vi "FTW-Scripter-Core_Process.vi"(0 "FTW Actor Instance Configuration":string="{\n  \"Identity\": \"FTW Scripter\",\n  \"InboxAddress\": \"inproc://*\",\n  \"LoggerAddress\": \"\",\n  \"Connections\": {},\n  \"Publishers\": {\n    \"ScripterStatus\": \"inproc://*\"\n  },\n  \"Subscriptions\": {},\n  \"Step Name Dictionary\": {},\n  \"Refresh Period\": 0.1\n}", 11 "ErrorIn":errorcluster) -> (15 "Error":errorcluster)   [LabVIEW 2015, in "FTW-Scripter-Core.lvclass"]
uses:
  FTW-Scripter-Core.lvclass
  source/actor/Instance/FTW-ActorInstance.lvclass
  source/actor/Message/Request/FTW-Message-IncomingRequest.lvclass
  source/actor/Message/Base/FTW-Message.lvclass
  source/actor/Instance-Extended/FTW-ActorExtended.lvclass
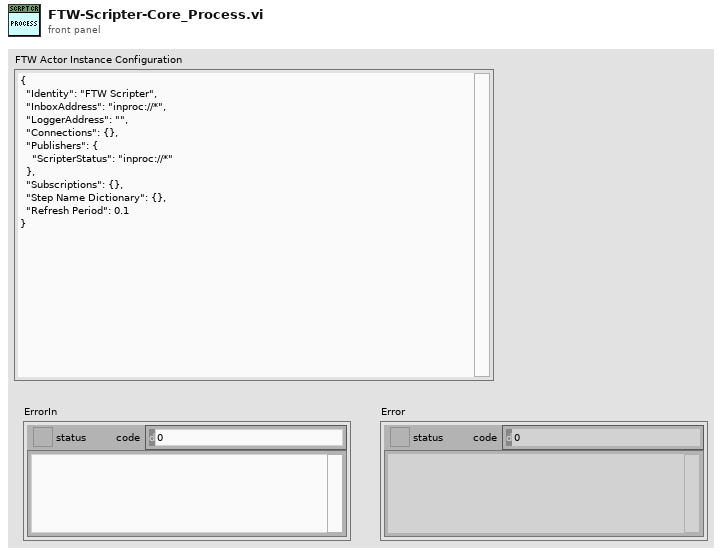
[diagram p1: front panel]
types:
  T1 = cluster{"Incoming Requests":refnum<event-registration>, "Local Messages":refnum<event-registration>, "Subscriber Registration":refnum<event-registration>}
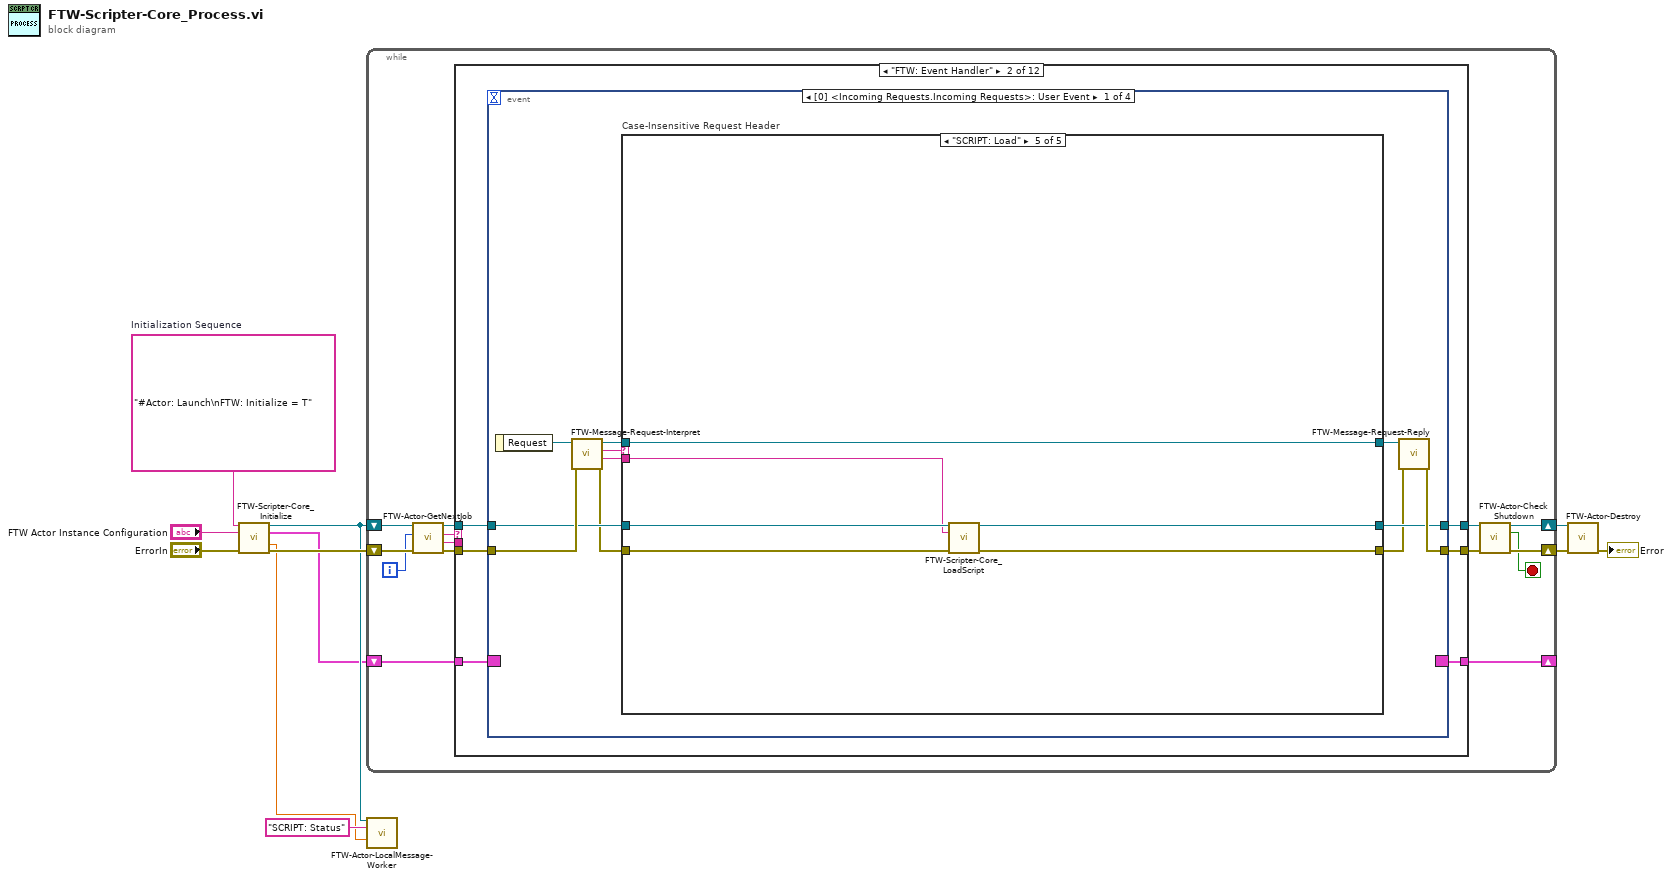
[diagram p0: block diagram]
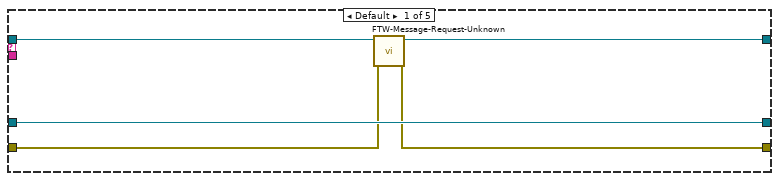
[diagram p3: hidden frame]
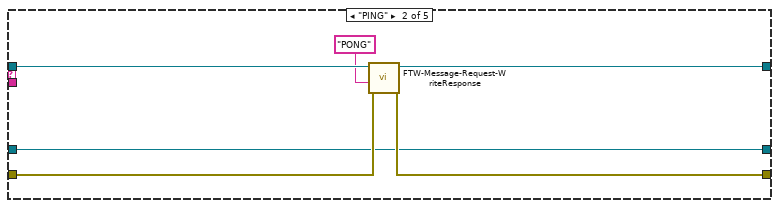
[diagram p4: hidden frame]
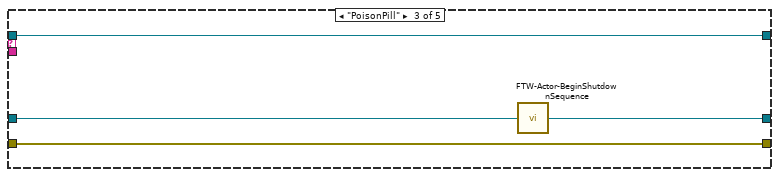
[diagram p5: hidden frame]
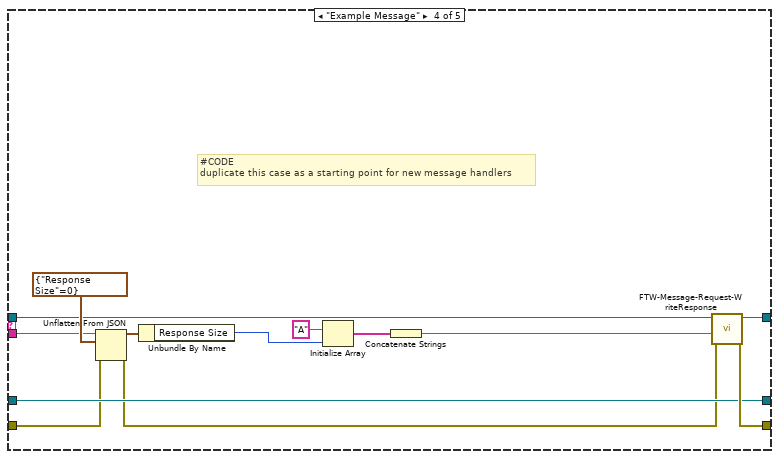
[diagram p6: hidden frame]
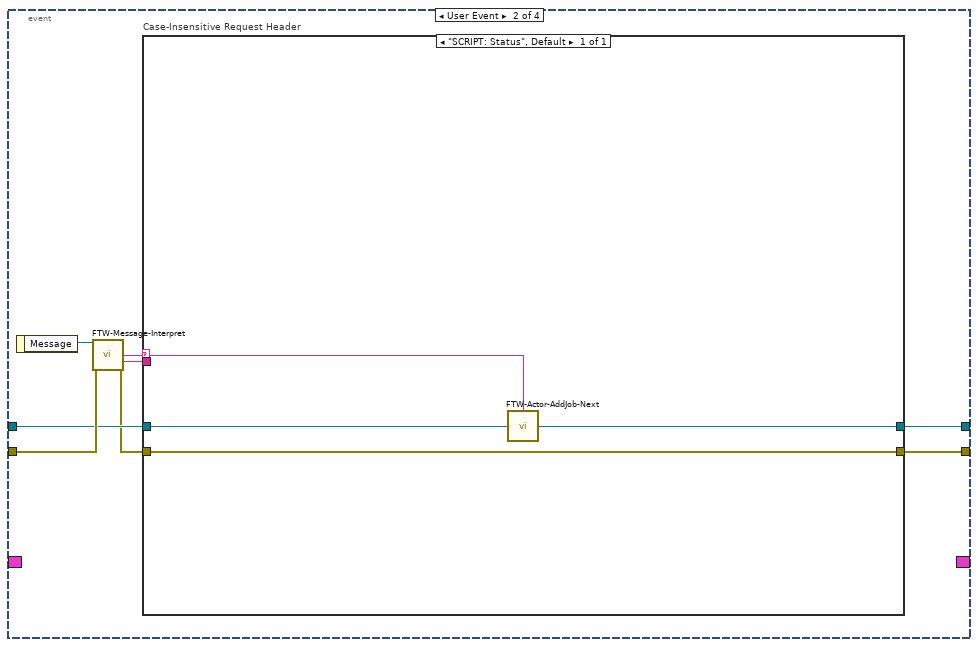
[diagram p7: hidden frame]
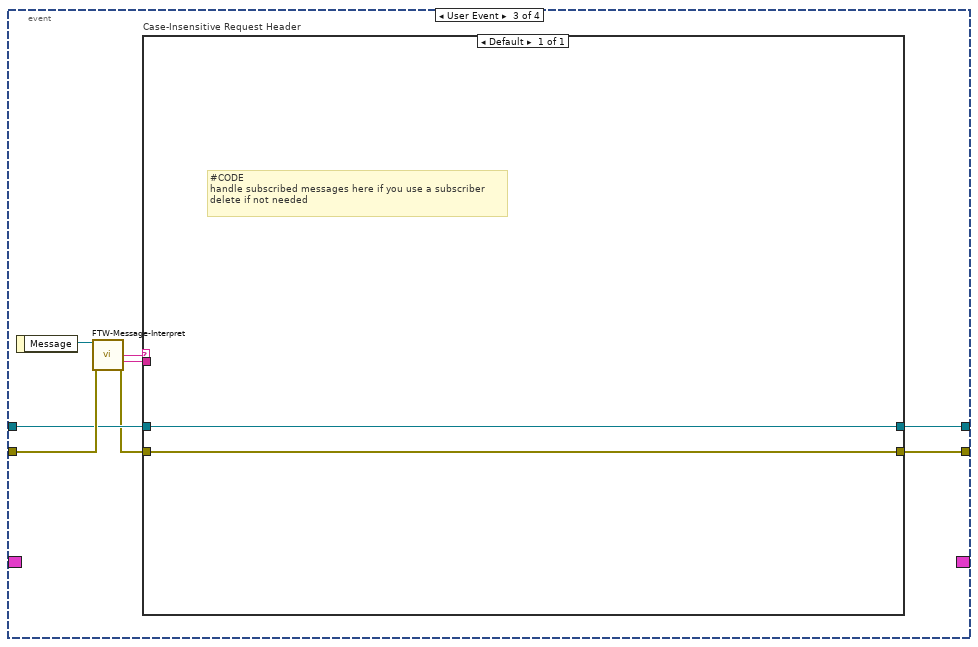
[diagram p8: hidden frame]
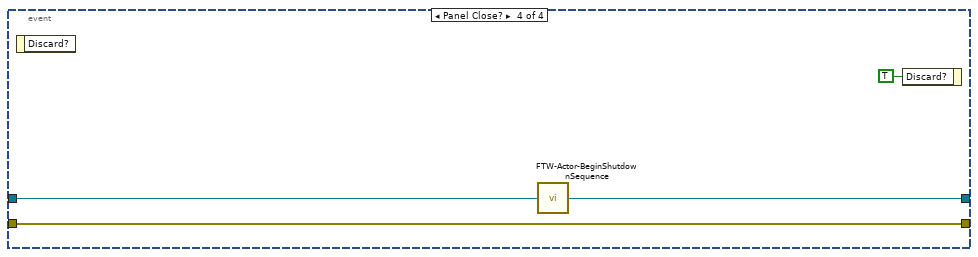
[diagram p9: hidden frame]
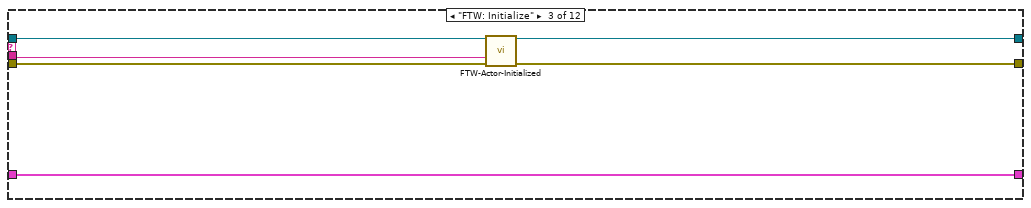
[diagram p10: hidden frame]
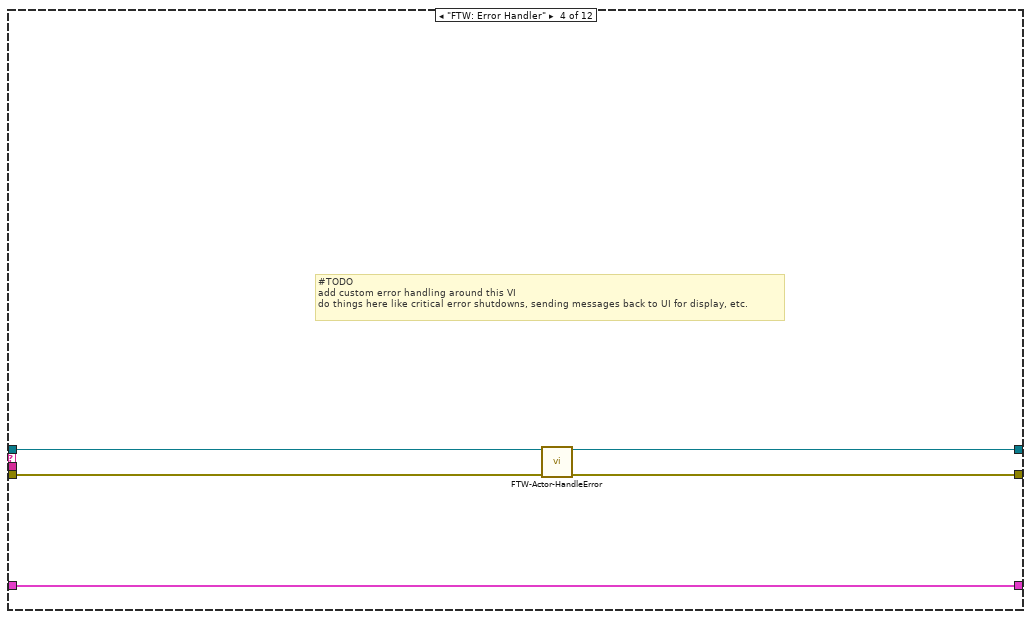
[diagram p11: hidden frame]
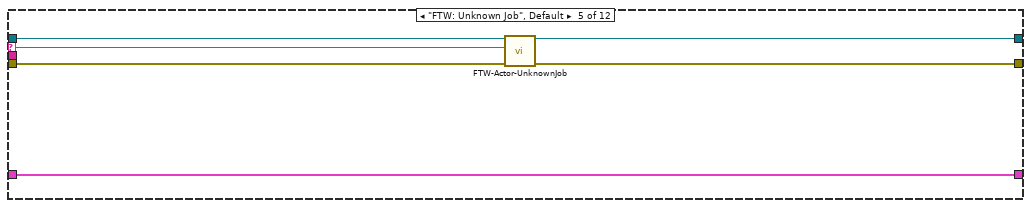
[diagram p12: hidden frame]
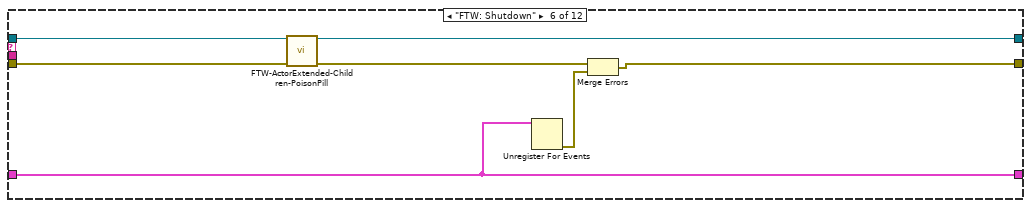
[diagram p13: hidden frame]
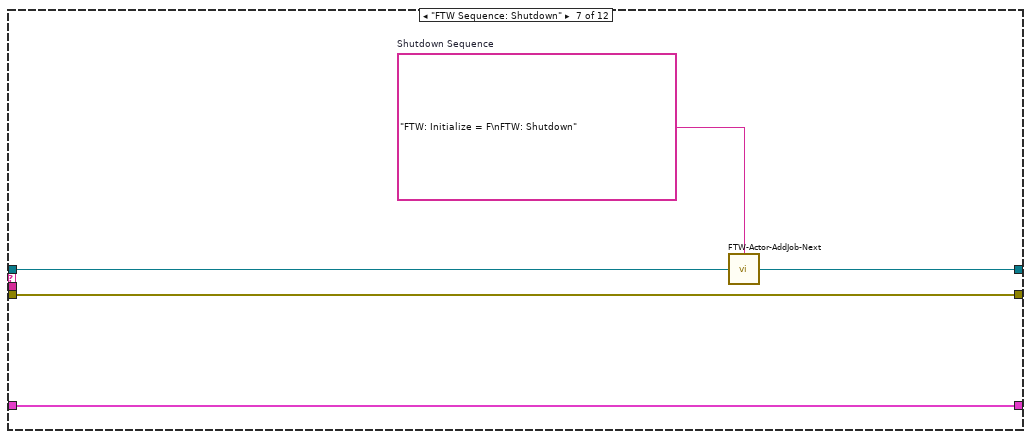
[diagram p14: hidden frame]
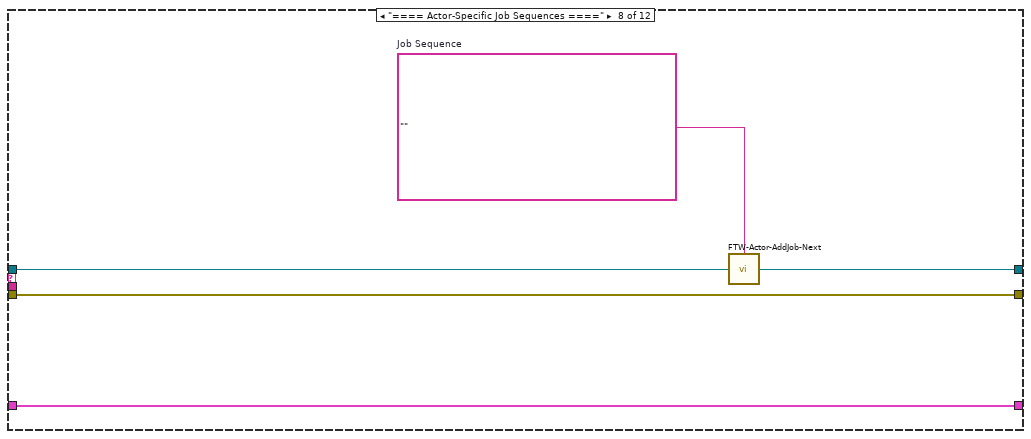
[diagram p15: hidden frame]
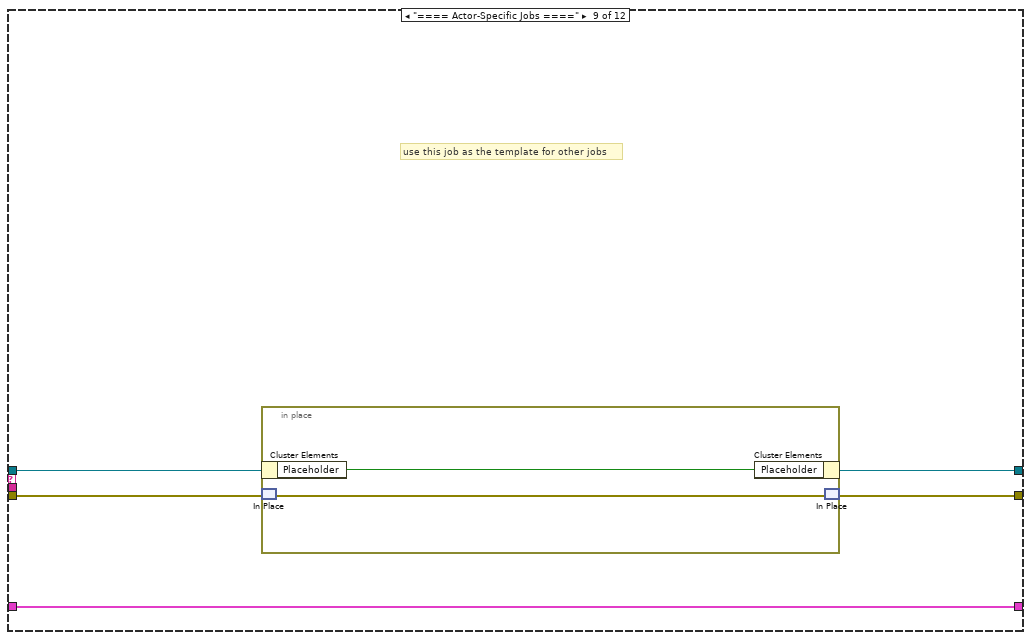
[diagram p16: hidden frame]
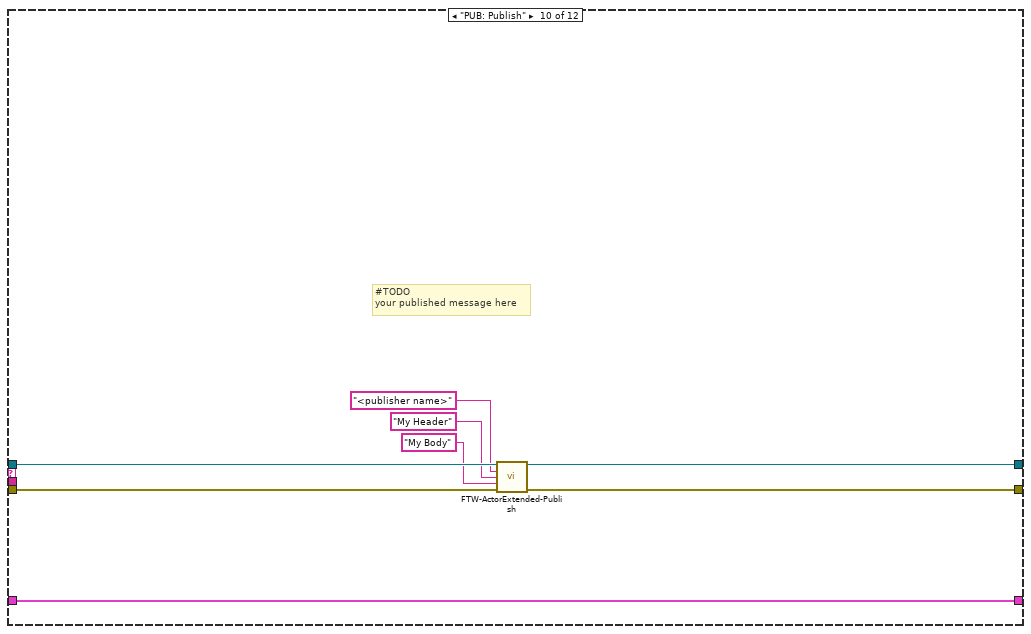
[diagram p17: hidden frame]
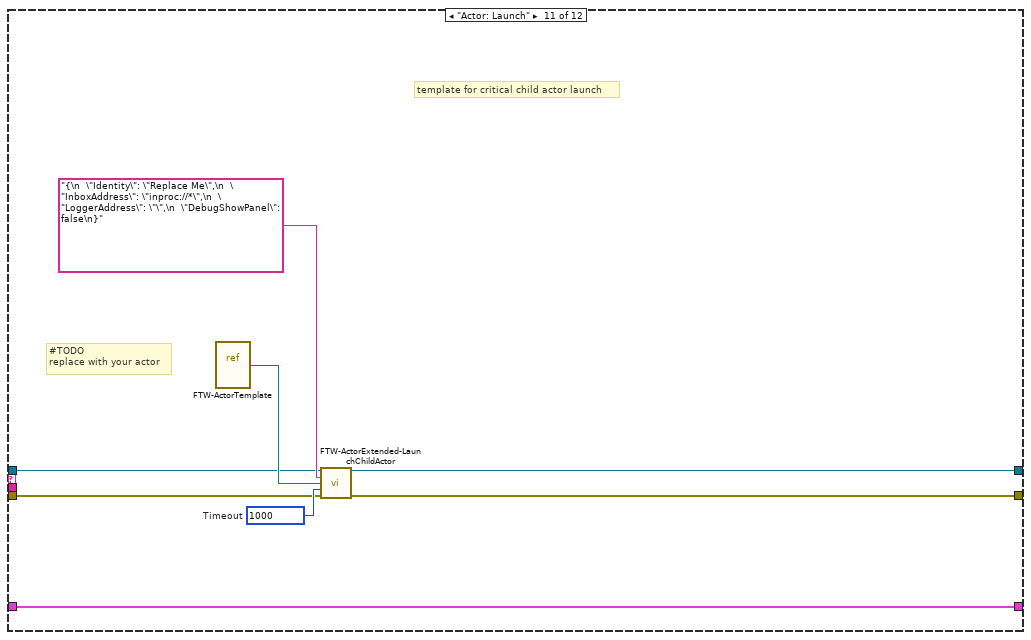
[diagram p18: hidden frame]
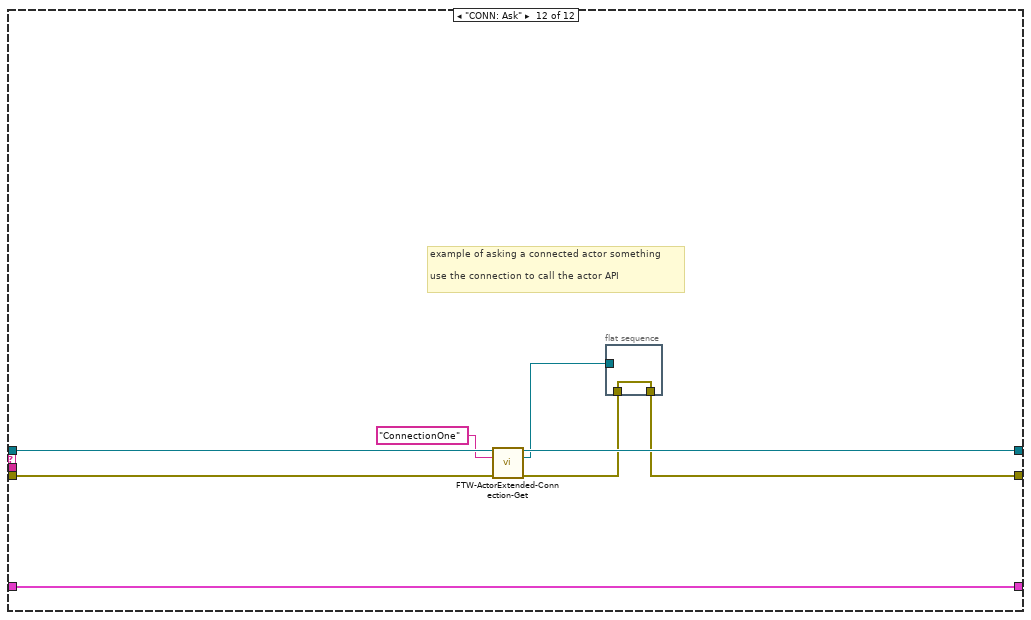
[diagram p19: hidden frame]
diagram:
  w7 = "#Actor: Launch\nFTW: Initialize = T"  # Initialization Sequence
  n1 = call "FTW-Scripter-Core_Initialize.vi"("Initialization Sequence"=w7, "FTW Actor Instance Configuration"="FTW Actor Instance Configuration", "error in (no error)"="ErrorIn") -> ("Actor Template-Core out"=w3:refnum<class "FTW-Scripter-Core.lvclass">, "Event Refnums"=w1:T1, "Refresh Period"=w2:dbl, "error out"=w8:errorcluster)  [unwired: 9 in]
  n2 = while {
    shift-right: [w15] -> w10
    shift-left: w8 -> [w22]
    shift-right: [w12] -> _
    shift-left: w1 -> [w25]
    shift-right: [w17] -> w11
    shift-left: w3 -> [w24]
    i -> [w13]
    stop <- w14 stop-if-true
    n3 = call "FTW-Actor-GetNextJob.vi"("error in"=w22, "Jobs Performed"=w13, "FTW Actor Instance"=w24) -> ("error out"=w21:errorcluster, "Job Data"=w19:string, "Job Name"=w20:string, "FTW Actor Instance out"=w23:refnum<class "FTW-Scripter-Core.lvclass">)  [unwired: 5 in]
    n4 = case shown="\"FTW: Event Handler\"" w20 {
      selector: w20 -> [_ _ _ _ w117 _ _ _ _ _ _ _]
      tunnel: [w27 w34 w108 w112 w120 w128 w133 w138 w142 w152 w157 w163] -> w16
      tunnel: w21 -> [w27 w33 w110 w114 w121 w129 w133 w138 w143 w153 w158 w169]
      tunnel: w25 -> [w28 w29 w111 w116 w122 w126 w134 w139 w144 w154 w162 w170]
      tunnel: [w28 w32 w111 w116 w122 w126 w134 w139 w144 w154 w162 w170] -> w12
      tunnel: w19 -> [_ _ w106 _ _ _ _ _ _ _ _ _]
      tunnel: [w26 w31 w109 w113 w118 w123 w131 w136 w140 w150 w155 w167] -> w18
      tunnel: w23 -> [w26 w30 w107 w115 w119 w124 w132 w137 w141 w151 w156 w168]
      frame "==== Featherweight Framework Jobs ====" {
      }
      frame "FTW: Event Handler" {
        n5 = event shown="[0] <Incoming Requests.Incoming Requests>: User Event" {
          selector: w29 -> [_ _ _ _]
          dyn-events: [_ _ _ _] -> w32
          timeout: _ -> [_ _ _ _]
          tunnel: [w44 w82 w94 w104] -> w34
          tunnel: w33 -> [w43 w86 w98 w104]
          tunnel: [w38 w83 w95 w102] -> w31
          tunnel: w30 -> [w42 w85 w97 w103]
          event User Event {
            n6 = event-data() -> ("Request"=w45:refnum<class "FTW-Message-IncomingRequest.lvclass">)  [unwired: 1 in]
            n7 = call "FTW-Message-Request-Interpret.vi"("error in"=w43, "FTW Incoming Request"=w45) -> ("error out"=w41:errorcluster, "Request Body"=w35:string, "Request Header"=w39:string, "FTW Incoming Request out"=w40:refnum<class "FTW-Message-IncomingRequest.lvclass">)  [unwired: 6 in]
            n8 = case "Case-Insensitive Request Header" shown="\"SCRIPT: Load\"" w39 {
              tunnel: [w48 w54 w59 w73 w75] -> w37
              tunnel: w41 -> [w49 w55 w59 w62 w76]
              tunnel: [w50 w53 w60 w71 w77] -> w38
              tunnel: w42 -> [w50 w53 w58 w71 w78]
              tunnel: w40 -> [w47 w56 w57 w63 w79]
              tunnel: [w46 w52 w57 w72 w79] -> w36
              tunnel: w35 -> [_ _ _ w61 w74]
              frame Default {
                n9 = call "FTW-Message-Request-Unknown.vi"("error in"=w49, "FTW Incoming Request"=w47) -> ("error out"=w48:errorcluster, "FTW Incoming Request Out"=w46:refnum<class "FTW-Message-IncomingRequest.lvclass">)  [unwired: 8 in]
              }
              frame "PING" {
                n10 = call "FTW-Message-Request-WriteResponse.vi"("error in"=w55, "Response Body"="PONG" ("Response Header"), "FTW Incoming Request"=w56) -> ("error out"=w54:errorcluster, "FTW Incoming Request out"=w52:refnum<class "FTW-Message-IncomingRequest.lvclass">)  [unwired: 7 in]
              }
              frame "PoisonPill" {
                n11 = call "FTW-Actor-BeginShutdownSequence.vi"("FTW Actor Instance"=w58) -> ("FTW Actor Instance out"=w60:refnum<class "FTW-Scripter-Core.lvclass">)  [unwired: 3 in]
              }
              frame "Example Message" {
                # "#CODE\nduplicate this case as a starting point for new message handlers"
                n12 = Unflatten From JSON(JSON string=w61, type and defaults=cluster{"Response Size":i32} {"Response Size"=0}, error in (no error)=w62) -> (value=w68:cluster{"Response Size":i32}, error out=w70:errorcluster)  [unwired: 4 in]
                n13 = Unbundle By Name(w68) -> ("Response Size"=w67:i32)
                n14 = Initialize Array("A", w67) -> (w65:string[])
                n15 = Concatenate Strings(w65) -> (w64:string)
                n16 = call "FTW-Message-Request-WriteResponse.vi"("error in"=w70, "Response Body"=w64, "FTW Incoming Request"=w63) -> ("error out"=w73:errorcluster, "FTW Incoming Request out"=w72:refnum<class "FTW-Message-IncomingRequest.lvclass">)  [unwired: 7 in]
              }
              frame "SCRIPT: Load" {
                n17 = call "FTW-Scripter-Core_LoadScript.vi"("FTW-Scripter-Core In"=w78, "Script"=w74, "error in"=w76) -> ("FTW-Scripter-Core Out"=w77:refnum<class "FTW-Scripter-Core.lvclass">, "error out"=w75:errorcluster)  [unwired: 11 in]
              }
            }
            n18 = call "FTW-Message-Request-Reply.vi"("FTW: Reply Error"=w37, "FTW Incoming Request"=w36) -> ("error out"=w44:errorcluster)  [unwired: 8 in, 1 out]
          }
          event User Event {
            n19 = event-data() -> ("Message"=w87:refnum<class "FTW-Message.lvclass">)  [unwired: 1 in]
            n20 = call-dynamic "FTW-Message-Interpret.vi"("FTW Message"=w87, "error in"=w86) -> ("Message Header"=w81:string, "Message Body"=w80:string, "error out"=w84:errorcluster)  [unwired: 9 in, 2 out]
            n21 = case "Case-Insensitive Request Header" shown="\"SCRIPT: Status\", Default" w81 {
              selector: w81 -> [w88]
              tunnel: [w90] -> w82
              tunnel: w84 -> [w90]
              tunnel: [w89] -> w83
              tunnel: w85 -> [w91]
              tunnel: w80 -> [_]
              frame "SCRIPT: Status", Default {
                n22 = call "FTW-Actor-AddJob-Next.vi"("Add Next in Job Queue"=w88, "FTW Actor Instance"=w91) -> ("FTW Actor Instance out"=w89:refnum<class "FTW-Scripter-Core.lvclass">)  [unwired: 2 in]
              }
            }
          }
          event User Event {
            n23 = event-data() -> ("Message"=w99:refnum<class "FTW-Message.lvclass">)  [unwired: 1 in]
            n24 = call-dynamic "FTW-Message-Interpret.vi"("FTW Message"=w99, "error in"=w98) -> ("Message Header"=w93:string, "Message Body"=w92:string, "error out"=w96:errorcluster)  [unwired: 9 in, 2 out]
            n25 = case "Case-Insensitive Request Header" shown="Default" w93 {
              tunnel: [w100] -> w94
              tunnel: w96 -> [w100]
              tunnel: [w101] -> w95
              tunnel: w97 -> [w101]
              tunnel: w92 -> [_]
              frame Default {
                # "#CODE\nhandle subscribed messages here if you use a subscriber\ndelete if not needed"
              }
            }
          }
          event Panel Close? {
            n26 = event-data() -> ()  [unwired: 1 in, 1 out]
            n27 = call "FTW-Actor-BeginShutdownSequence.vi"("FTW Actor Instance"=w103) -> ("FTW Actor Instance out"=w102:refnum<class "FTW-Scripter-Core.lvclass">)  [unwired: 3 in]
            n28 = event-data("Discard?"=TRUE) -> ()  [unwired: 1 in, 1 out]
          }
        }
      }
      frame "FTW: Initialize" {
        n29 = call-dynamic "FTW-Actor-Initialized.vi"("FTW Actor Instance"=w107, "Positive Init?"=w106, "error in"=w110) -> ("FTW Actor Instance out"=w109:refnum<class "FTW-Scripter-Core.lvclass">, "error out"=w108:errorcluster)  [unwired: 11 in]
      }
      frame "FTW: Error Handler" {
        # "#TODO\nadd custom error handling around this VI\ndo things here like critical error shutdowns, sending messages back to UI for display, etc."
        n30 = call-dynamic "FTW-Actor-HandleError.vi"("FTW Actor Instance"=w115, "error in"=w114) -> ("FTW Actor Instance out"=w113:refnum<class "FTW-Scripter-Core.lvclass">, "error out"=w112:errorcluster)  [unwired: 10 in, 2 out]
      }
      frame "FTW: Unknown Job", Default {
        n31 = call-dynamic "FTW-Actor-UnknownJob.vi"("FTW Actor Instance"=w119, "Unknown Job"=w117, "error in"=w121) -> ("FTW Actor Instance out"=w118:refnum<class "FTW-Scripter-Core.lvclass">, "error out"=w120:errorcluster)  [unwired: 11 in]
      }
      frame "FTW: Shutdown" {
        n32 = call "FTW-ActorExtended-Children-PoisonPill.vi"("FTW-ActorExtended In"=w124, "error in"=w129) -> ("FTW-ActorExtended Out"=w123:refnum<class "FTW-Scripter-Core.lvclass">, "error out"=w125:errorcluster)  [unwired: 12 in]
        n33 = Unregister For Events(event registration refnum=w126) -> (error out=w127:errorcluster)  [unwired: 1 in]
        n34 = Merge Errors(w125, w127) -> (w128:errorcluster)
      }
      frame "FTW Sequence: Shutdown" {
        w130 = "FTW: Initialize = F\nFTW: Shutdown"  # Shutdown Sequence
        n35 = call "FTW-Actor-AddJob-Next.vi"("Add Next in Job Queue"=w130, "FTW Actor Instance"=w132) -> ("FTW Actor Instance out"=w131:refnum<class "FTW-Scripter-Core.lvclass">)  [unwired: 2 in]
      }
      frame "==== Actor-Specific Job Sequences ====" {
        w135 = ""  # Job Sequence
        n36 = call "FTW-Actor-AddJob-Next.vi"("Add Next in Job Queue"=w135, "FTW Actor Instance"=w137) -> ("FTW Actor Instance out"=w136:refnum<class "FTW-Scripter-Core.lvclass">)  [unwired: 2 in]
      }
      frame "==== Actor-Specific Jobs ====" {
        # "use this job as the template for other jobs"
        n37 = in-place {
          n38 = in-place-cluster #1(w141) -> ("Placeholder"=w145:bool)
          n39 = in-place-match #2(w143) -> (w146:errorcluster)
          n40 = in-place-cluster #1("Placeholder"=w145) -> (w140:refnum<class "FTW-Scripter-Core.lvclass">)
          n41 = in-place-match #2(w146) -> (w142:errorcluster)
        }
      }
      frame "PUB: Publish" {
        # "#TODO\nyour published message here"
        n42 = call "FTW-ActorExtended-Publish.vi"("FTW-ActorExtended In"=w151, "Publisher Name"="<publisher name>", "Message Header"="My Header" ("Header"), "Message Body"="My Body" ("Header"), "error in"=w153) -> ("FTW-ActorExtended Out"=w150:refnum<class "FTW-Scripter-Core.lvclass">, "error out"=w152:errorcluster)  [unwired: 9 in]
      }
      frame "Actor: Launch" {
        w161 = 1000  # Timeout
        # "#TODO\nreplace with your actor"
        # "template for critical child actor launch"
        n43 = vi-ref "FTW-ActorTemplate.vi"() -> (w160:refnum<vi>)
        n44 = call "FTW-ActorExtended-LaunchChildActor.vi"("FTW Actor Connector Type"=w156, "Configuration"="{\n  \"Identity\": \"Replace Me\",\n  \"InboxAddress\": \"inproc://*\",\n  \"LoggerAddress\": \"\",\n  \"DebugShowPanel\": false\n}", "Actor VI Refnum"=w160, "Timeout"=w161, "error in"=w158) -> ("FTW-ActorExtended.lvclass"=w155:refnum<class "FTW-Scripter-Core.lvclass">, "error out"=w157:errorcluster)  [unwired: 6 in, 3 out]
      }
      frame "CONN: Ask" {
        # "example of asking a connected actor something\n\nuse the connection to call the actor API"
        n45 = call "FTW-ActorExtended-Connection-Get.vi"("FTW-ActorExtended In"=w168, "Connector Name"="ConnectionOne" ("Publisher Name"), "error in"=w169) -> ("FTW-ActorExtended Out"=w167:refnum<class "FTW-Scripter-Core.lvclass">, "FTW Actor Connector"=w165:refnum<class "FTW-ActorConnector.lvclass">, "error out"=w164:errorcluster)  [unwired: 10 in]
        n46 = flat-sequence {
          tunnel: w165 -> [_]
          tunnel: w164 -> [w171]
          tunnel: [w171] -> w163
          frame #0 {
          }
        }
      }
    }
    n47 = call "FTW-Actor-CheckShutdown.vi"("FTW Actor Instance"=w18, "error in"=w16) -> ("FTW Actor Instance out"=w17:refnum<class "FTW-Scripter-Core.lvclass">, "Shutdown?"=w14:bool, "error out"=w15:errorcluster)  [unwired: 11 in]
  }
  n48 = call-dynamic "FTW-Actor-LocalMessage-Worker.vi"("FTW-ActorInstance In"=w3, "Message Header"="SCRIPT: Status", "Send Rate"=w2) -> ()  [unwired: 13 in]
  n49 = call-dynamic "FTW-Actor-Destroy.vi"("FTW Actor Instance"=w11, "error in"=w10) -> ("error out"=→"Error":errorcluster)  [unwired: 13 in]
